vi "Get Test Parameter.vi"(7 "Data Value ID":string, 8 "error in (no error)":errorcluster, 11 "Test in":refnum<class "Test.lvclass">) -> (0 "error out":errorcluster, 1 "Data Type":T1, 2 "Test Parameter":string)   [LabVIEW 2018, in "Test.lvclass"]
doc: "Pulls the test parameter specified by Data Value ID and formats it to a string. Also outputs the data type to aid parsing back to the correct value"
uses:
  Test.lvclass
  <vilib>/Utility/Data Type/Type Definitions/Data Type.ctl
  Test.lvclass/Test.ctl
  a187ca40-752b-45be-9709-565cb8855a9a.vi
  229dbb40-5538-4285-934d-f803a1a9958d.vi
  <vilib>/JDP Science/JSONtext/String Subset.vi
  <vilib>/JDP Science/JSONtext/Parsing/Parse Full Path or Item Name.vi
  <vilib>/JDP Science/JSONtext/Offset/Find Item Locations by Path.vi
  <vilib>/JDP Science/JSONtext/JSON text to Variant.vi
  <vilib>/Utility/Data Type/NI_Data Type.lvlib
  <vilib>/JDP Science/JSONtext/JSONtext.lvlib
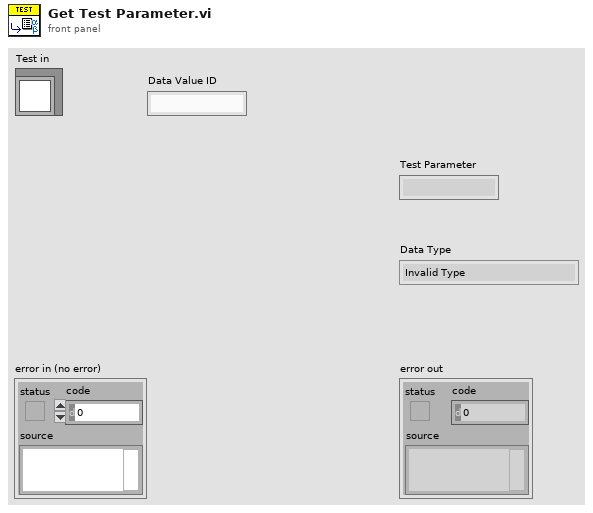
[diagram p1: front panel]
types:
  T1 = typedef "NI_Data Type.lvlib/Data Type.ctl" = enum8{"Invalid Type", "Void", "I8", "I16", "I32", "I64", "U8", "U16", "U32", "U64", "Single Float", "Double Float", "Extended Float", "Single Complex", "Double Complex", "Extended Complex", "Enum U8", "Enum U16", "Enum U32", "Enum U64", "Single Float With Unit", "Double Float With Unit", "Extended Float With Unit", "Single Complex with Unit", "Double Complex with Unit", "Extended Complex with Unit", "Boolean", "String", "Path", "Picture", "Tag", "Array", "Cluster", "Variant", "LV Variant", "Waveform", "Timestamp", "Digital Waveform", "Digital Data", "ExpressData", "Refnum", "External Data", "VI", "Poly VI", "LabVIEW Class Instance", "Fixed Point"}
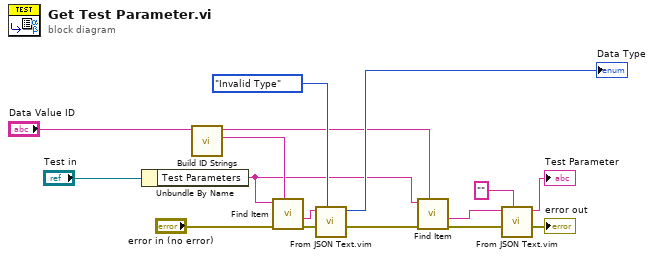
[diagram p0: block diagram]
diagram:
  n1 = Unbundle By Name("Test in") -> ("Test Parameters"=w6:string)
  n2 = call "Build ID Strings.vi"("Data Value ID"="Data Value ID") -> ("Type ID"=w14:string, "Value ID"=w7:string)  [unwired: 9 in]
  n3 = call <vilib>:"Find Item.vi"("$Path or Item Name"=w14, "error in (no error)"="error in (no error)", "JSON"=w6) -> ("error out"=w12:errorcluster, "<JSON>"=w13:string)  [unwired: 5 in, 2 out]
  n4 = call "From JSON Text.vim"("Data Type and Default Value"=Data_Type."Invalid Type" ("Data Type"), "error in (no error)"=w12, "JSON"=w13) -> ("error out"=w5:errorcluster, "Data out"=→"Data Type":T1)  [unwired: 7 in]
  n5 = call <vilib>:"Find Item.vi"("$Path or Item Name"=w7, "error in (no error)"=w5, "JSON"=w6) -> ("error out"=w9:errorcluster, "<JSON>"=w8:string)  [unwired: 5 in, 2 out]
  n6 = call "From JSON Text.vim"("Data Type and Default Value"="", "error in (no error)"=w9, "JSON"=w8) -> ("error out"=→"error out":errorcluster, "Data out"=→"Test Parameter":string)  [unwired: 7 in]
